vi "Serialize as XML.vi"(8 "error in (no error)":errorcluster, 11 "Data Item in":refnum<class "Data Item.lvclass">) -> (0 "error out":errorcluster, 2 "XML Fragment":string, 3 "Data Item out":refnum<class "Data Item.lvclass">)   [LabVIEW 2018, in "VILab.lvlib" / "Data Item.lvclass"]
uses:
  Data Item.lvclass
  Data Item.lvclass/Data Item.ctl
  VILab.lvlib
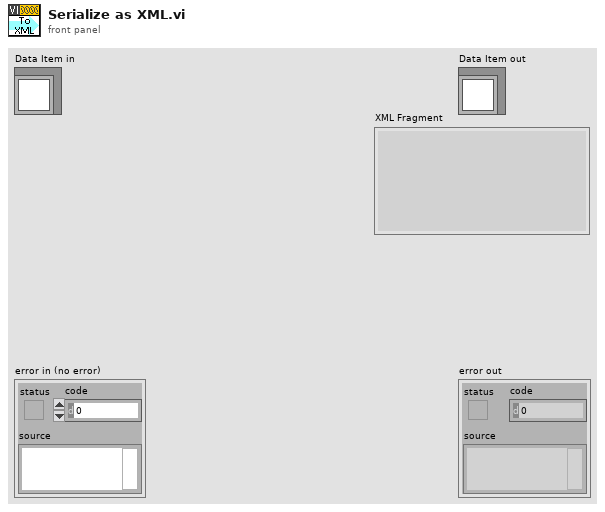
[diagram p1: front panel]
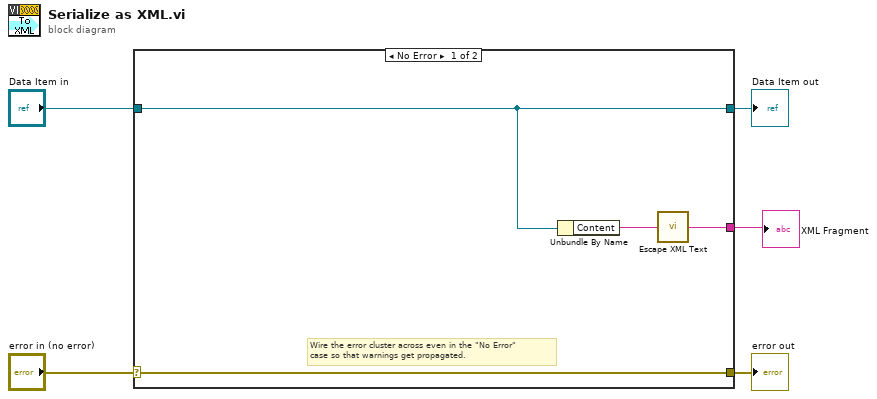
[diagram p0: block diagram]
diagram:
  n1 = case shown="No Error" "error in (no error)" {
    selector: "error in (no error)" -> [w9 w11]
    tunnel: [w9 w11] -> w4
    tunnel: [w8 w10] -> w2
    tunnel: "Data Item in" -> [w8 w10]
    tunnel: [w6 _] -> w1
    frame No Error {
      # "Wire the error cluster across even in the \"No Error\"\ncase so that warnings get propagated."
      n2 = Unbundle By Name(w8) -> ("Content"=w7:string)
      n3 = call "Escape XML Text.vi"("String"=w7) -> ("Escaped"=w6:string)
    }
    frame Error {
    }
  }
  "error out" <- w4
  "Data Item out" <- w2
  "XML Fragment" <- w1
